vi "Digital Pattern Gen 1.0 Write Inputs.vi"(5 "Device inputs":dbl[](array[numeric]), 6 "offset convert":dbl, 7 "Last Device inputs":dbl[](array[numeric]), 8 "error in (no error)":errorcluster, 9 "input reference in":T1, 10 "input in":cluster{"Offset":i16}, 11 "FIFO indexes.inputs":T2) -> (0 "error out":errorcluster, 1 "input reference out":T1, 2 "input out":cluster{"Offset":i16})   [LabVIEW 2015, in "Engine Simulation Toolkit Engine.lvlib"]
uses:
  Engine Simulation Toolkit Engine.lvlib
  Shared/1.0 Digital Pattern Gen FIFO Idxs.ctl
  Digital Pattern Gen 1.0 Input Ref.ctl
  Shared/Engine Simulation Toolkit Shared.lvlib
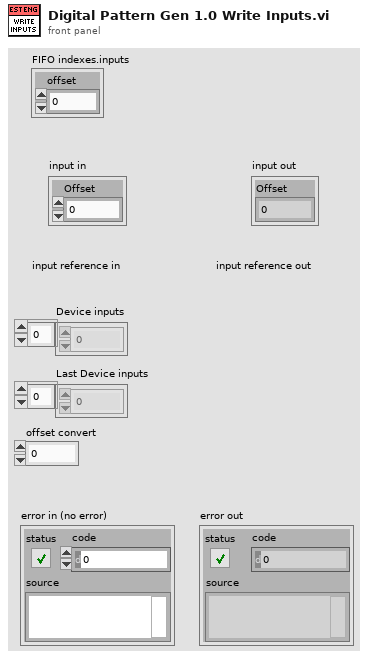
[diagram p1: front panel]
types:
  T1 = typedef "Engine Simulation Toolkit Engine.lvlib/Digital Pattern Gen 1.0 Input Ref.ctl" = refnum<k20>
  T2 = typedef "Engine Simulation Toolkit Shared.lvlib/1.0 Digital Pattern Gen FIFO Idxs.ctl" = cluster{"offset":i32}
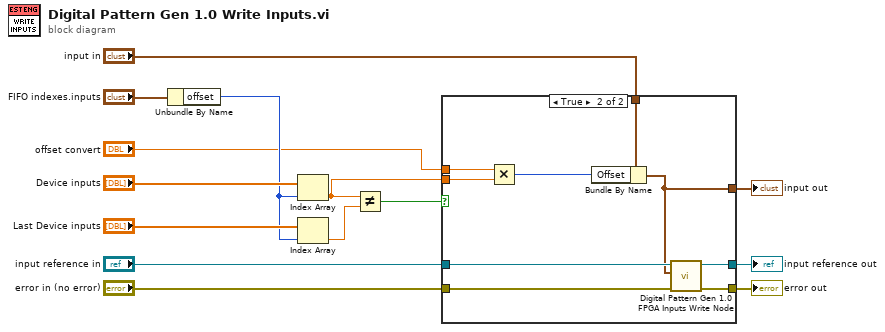
[diagram p0: block diagram]
diagram:
  n1 = Unbundle By Name("FIFO indexes.inputs") -> ("offset"=w6:i32)
  n2 = Index Array(array="Device inputs", index=w6) -> (element=w3:dbl)
  n3 = Index Array(array="Last Device inputs", index=w6) -> (element=w4:dbl)
  n4 = Not Equal?(x=w3, y=w4) -> (x != y?=w2:bool)
  n5 = case shown="True" w2 {
    tunnel: "error in (no error)" -> [w15 w26]
    tunnel: "input reference in" -> [w16 w25]
    tunnel: [w15 w24] -> w12
    tunnel: [w16 w23] -> w11
    tunnel: "input in" -> [w17 w22]
    tunnel: [w17 w21] -> w5
    tunnel: w3 -> [_ w20]
    tunnel: "offset convert" -> [_ w19]
    frame False {
    }
    frame True {
      n6 = Multiply(x=w19, y=w20) -> (x*y=w18:i16)
      n7 = Bundle By Name(cluster=w22, "Offset"=w18) -> (w21:cluster{"Offset":i16})
      n8 = call "Digital Pattern Gen 1.0 FPGA Inputs Write Node.vi"("error in (no error)"=w26, "input in"=w21, "Refnum in"=w25) -> ("error out"=w24:errorcluster, "Refnum out"=w23:T1)  [unwired: 7 in]
    }
  }
  "error out" <- w12
  "input out" <- w5
  "input reference out" <- w11
